vi "Read VI refs.vi"(8 "error in (no error)":errorcluster, 11 "Control in":refnum<class "Control-Server.lvclass">) -> (0 "error out":errorcluster, 2 "VI refs":refnum<vi>[](array[refnum]), 3 "Control out":refnum<class "Control-Server.lvclass">)   [LabVIEW 2019, in "Control-Server.lvclass"]
uses:
  Control-Server.lvclass
  Control-Server.lvclass/Control-Server.ctl
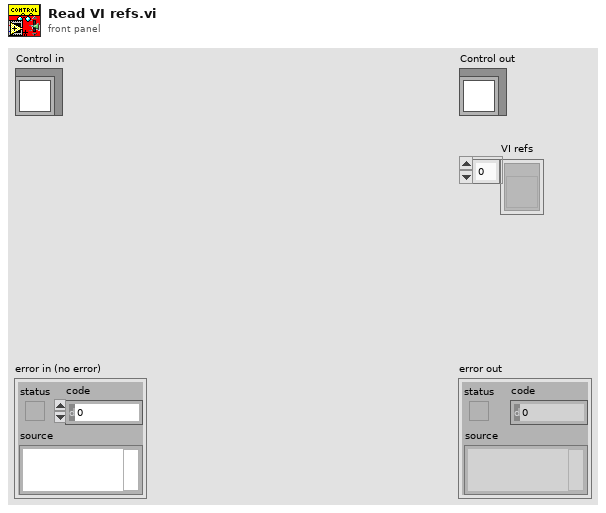
[diagram p1: front panel]
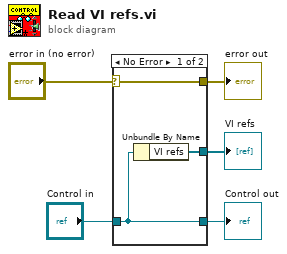
[diagram p0: block diagram]
diagram:
  n1 = case shown="No Error" "error in (no error)" {
    selector: "error in (no error)" -> [w8 w9]
    tunnel: [w8 w9] -> w4
    tunnel: [w7 w10] -> w2
    tunnel: "Control in" -> [w7 w10]
    tunnel: [w6 _] -> w1
    frame No Error {
      n2 = Unbundle By Name(w7) -> ("VI refs"=w6:refnum<vi>[])
    }
    frame Error {
    }
  }
  "error out" <- w4
  "Control out" <- w2
  "VI refs" <- w1
